vi "DBM File Save.vi"(8 "에러 입력":errorcluster caption="에러 입력(에러 없음)", 11 "Table 입력":refnum<vi>) -> (0 "에러 출력":errorcluster, 3 "File path":path caption="경로 복제")   [LabVIEW 2020]
uses:
  Controls/Cmd_File path.ctl
  <vilib>/Utility/sysdir.llb/System Directory Type.ctl
  Controls/Cmd_File Type.ctl
  <vilib>/Utility/NIReport.llb/Report Type.ctl
  Public/Polymorph/Cell Space_Excel.vi
  <vilib>/Utility/NIReport.llb/NI_report.lvclass
  <vilib>/Utility/NIReport.llb/NI_ReportGenerationCore.lvlib
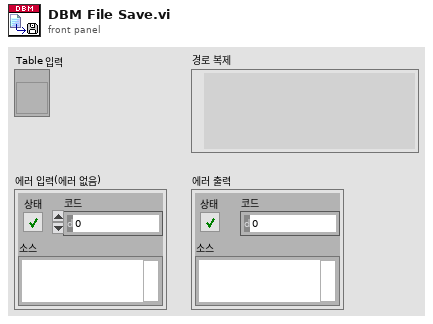
[diagram p1: front panel]
types:
  T1 = typedef "NI_ReportGenerationCore.lvlib/Report Type.ctl" = enum16{"HTML", "Word", "Excel"}
  T2 = typedef "Cmd_File Type.ctl" = enum16{"엑셀", "엑셀(2003)", "텍스트", "설정", "2진", "VI", "CSV", "LOG", "폴더"}
  T3 = typedef "System Directory Type.ctl" = i32
  T4 = typedef "Cmd_File path.ctl" = enum16{"에러로그", "데이터파일경로", "성적서원본", "지난성적서", "Data Files", "경로생성", "Updater", "Template", "설정파일경로", "FTP Upload", "Update 경로", "어플리케이션"}
  T5 = enum16{"maximized", "minimized", "normal", "no change"}
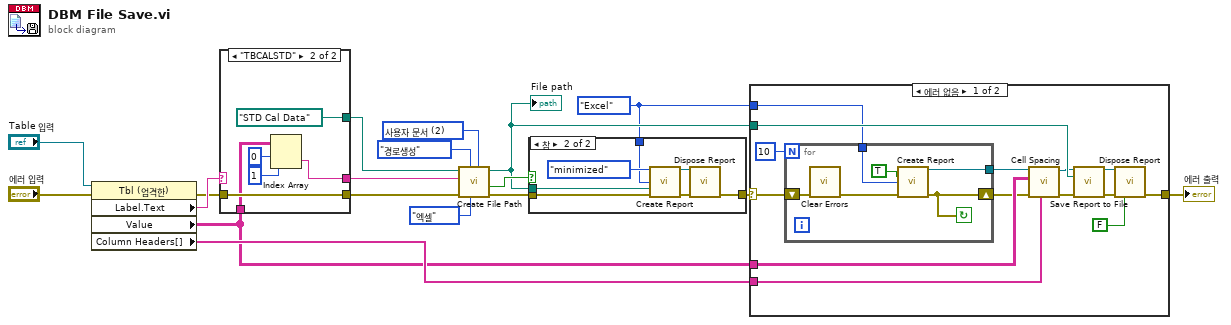
[diagram p0: block diagram]
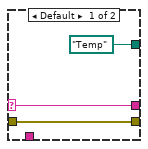
[diagram p4: hidden frame]
diagram:
  w1 = Report_Type."Excel" ("report type")
  w6 = T3 2 items=["사용자 홈"=0, "사용자 데스크탑"=1, "사용자 문서"=2, "사용자 어플리케이션 데이터"=3, "사용자 환경"=4, "사용자 임시"=5, "퍼블릭 문서"=6, "퍼블릭 어플리케이션 데이터"=7, "퍼블릭 환경"=8, "퍼블릭 캐시"=13, "시스템 코어 라이브러리"=9, "시스템 설치된 라이브러리"=10, "어플리케이션 파일"=11, "부팅 볼륨 루트"=12] ("system directory type")
  n1 = property class="Tbl (엄격한)"(reference="Table 입력", error in="에러 입력") -> (error out=w12:errorcluster, "Label.Text"=w14:string, "Value"=w11:string[][], "Column Headers[]"=w15:string[])  [unwired: 1 out]
  n2 = case shown="\"TBCALSTD\"" w14 {
    selector: w14 -> [w21 _]
    tunnel: [w21 w22] -> w5
    tunnel: [path "Temp" ("생성할 폴더") path "STD Cal Data" ("생성할 폴더")] -> w10
    tunnel: w12 -> [w19 w26]
    tunnel: [w19 w26] -> w9
    tunnel: w11 -> [_ w25]
    frame Default {
    }
    frame "TBCALSTD" {
      n3 = Index Array(array=w25, index (row)=0 ("인덱스 (행)"), index (col)=1 ("비활성화된 인덱스 (열)")) -> (element=w22:string)
    }
  }
  n4 = call "Create File Path.vi"("system directory type"=w6, "파일타입"=Cmd_File_Type."엑셀", "항목"=Cmd_File_path."경로생성", "에러 입력"=w9, "문자열 in"=w5, "폴더명 in"=w10) -> ("error out"=w8:errorcluster, "파일존재?"=w4:bool, "파일경로"=w3:path)  [unwired: 2 in, 1 out]
  "File path" <- w3
  n5 = case shown="참" w4 {
    tunnel: [w28 w33] -> w13
    tunnel: w8 -> [w28 w32]
    tunnel: w3 -> [_ w31]
    tunnel: w1 -> [_ w29]
    frame False {
    }
    frame True {
      n6 = call <vilib>:"Create Report.vi"("window state (normal)"=T5."minimized", "report type"=w29, "template (empty)"=w31, "error in (no error)"=w32) -> ("report out"=w35:refnum<class "NI_report.lvclass">, "error out"=w34:errorcluster)  [unwired: 10 in]
      n7 = call-dynamic "Dispose Report.vi"("report in"=w35, "error in (no error)"=w34) -> ("error out"=w33:errorcluster)  [unwired: 13 in]
    }
  }
  n8 = case shown="에러 없음" w13 {
    selector: w13 -> [w37 w56]
    tunnel: [w49 w56] -> w18
    tunnel: w3 -> [w48 _]
    tunnel: w1 -> [w47 _]
    tunnel: w15 -> [w44 _]
    tunnel: w11 -> [w39 _]
    frame No Error {
      n9 = for {
        N: 10 -> [_]
        tunnel: w47 -> [w55]
        tunnel: [w54] -> w40
        shift-right: [w50] -> w38
        shift-left: w37 -> [w52]
        stop <- w50 continue-if-true
        n10 = call <vilib>:"Clear Errors.vi"("error in (no error)"=w52) -> ("error out"=w51:errorcluster)  [unwired: 5 in, 1 out]
        n11 = call <vilib>:"Create Report.vi"("display alerts? (F)"=TRUE, "report type"=w55, "error in (no error)"=w51) -> ("report out"=w54:refnum<class "NI_report.lvclass">, "error out"=w50:errorcluster)  [unwired: 11 in]
      }
      n12 = call-poly "Cell Spacing.vi"("Col Header in"=w44, "error in"=w38, "Data in"=w39, "report in"=w40) -> ("error out"=w42:errorcluster, "report out"=w43:refnum<class "NI_report.lvclass">)  [unwired: 5 in, 1 out]
      n13 = call-dynamic "Save Report to File.vi"("report in"=w43, "report file path"=w48, "error in (no error)"=w42) -> ("report out"=w46:refnum<class "NI_report.lvclass">, "error out"=w45:errorcluster)  [unwired: 11 in]
      n14 = call-dynamic "Dispose Report.vi"("report in"=w46, "error in (no error)"=w45, "close report? (T)"=FALSE) -> ("error out"=w49:errorcluster)  [unwired: 12 in]
    }
    frame Error {
    }
  }
  "에러 출력" <- w18
